vi "UMB_ForebrainBehavior.vi"(8 "behavior weights":i8[](array[numeric]), 10 "Velocity":i8[](array[numeric]), 11 "Goodness":i8[](array[numeric])) -> (3 "Behavior Output":T1)   [LabVIEW 2012]
uses:
  NINJA Code/Tugboat/Robo_Programs/behaviorOutput_t.ctl
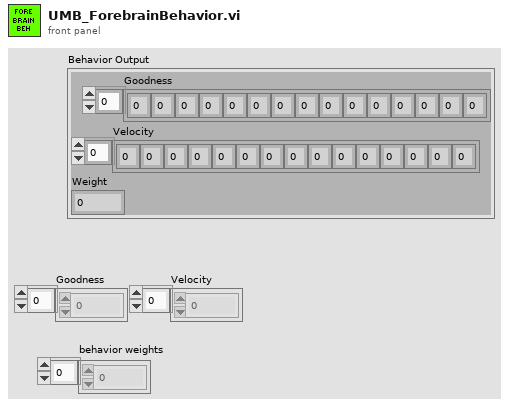
[diagram p1: front panel]
types:
  T1 = typedef "behaviorOutput_t.ctl" = cluster{"Goodness":i8[], "Velocity":i8[], "Weight":i8}
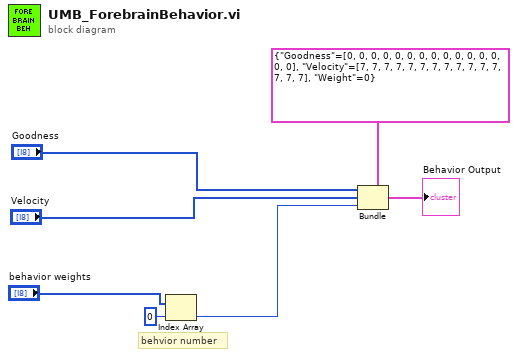
[diagram p0: block diagram]
diagram:
  # "behvior number"
  n1 = Index Array(array="behavior weights", index=0) -> (element=w5:i8)
  n2 = Bundle(cluster=T1 {"Goodness"=[0, 0, 0, 0, 0, 0, 0, 0, 0, 0, 0, 0, 0, 0, 0], "Velocity"=[7, 7, 7, 7, 7, 7, 7, 7, 7, 7, 7, 7, 7, 7, 7], "Weight"=0} ("Behavior Output"), "Goodness"="Goodness", "Velocity"="Velocity", "Weight"=w5) -> (→"Behavior Output":T1)
